vi "capture to clipboard.vi"(8 "error in (no error)":errorcluster, 11 "hwnd in":u32) -> (0 "error out":errorcluster, 3 "hwnd out":u32)   [LabVIEW 2011]
uses:
  user32.dll
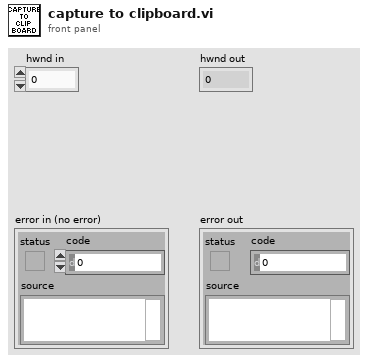
[diagram p1: front panel]
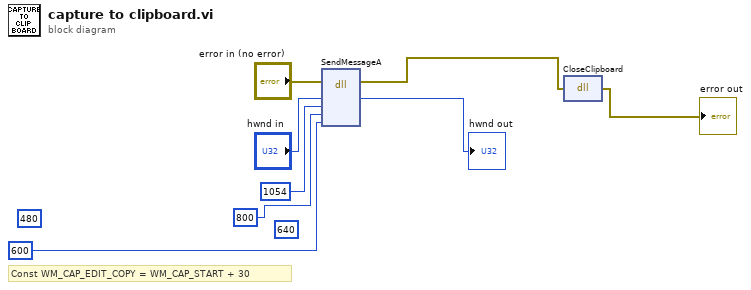
[diagram p0: block diagram]
diagram:
  (unwired) u32 480 ("lparam")
  (unwired) u32 640 ("wParam")
  # "Const WM_CAP_EDIT_COPY = WM_CAP_START + 30"
  n1 = dll-call lib="user32.dll" fn="SendMessageA"(error in="error in (no error)", "hwnd"="hwnd in", "msg"=u32 1054, "wParam"=u32 800, "lparam"=u32 600) -> (error out=w3:errorcluster, "hwnd"=→"hwnd out":u32)  [unwired: 6 in, 1 out]
  n2 = dll-call lib="user32.dll" fn="CloseClipboard"(error in=w3) -> (error out=→"error out":errorcluster)  [unwired: 3 in, 1 out]
